vi "Read acquisition start time (0.0 s).vi"(8 "error in (no error)":errorcluster, 11 "Configure Acquisition Record Msg in":refnum<class "Configure Acquisition Record Msg.lvclass">) -> (0 "error out":errorcluster, 2 "acquisition start time (0.0 s)":dbl[unit] format="%.3f", 3 "Configure Acquisition Record Msg out":refnum<class "Configure Acquisition Record Msg.lvclass">)   [LabVIEW 2015, in "CS++Scope.lvlib" / "Configure Acquisition Record Msg.lvclass"]
uses:
  Configure Acquisition Record Msg.lvclass
  Configure Acquisition Record Msg.lvclass/Configure Acquisition Record Msg.ctl
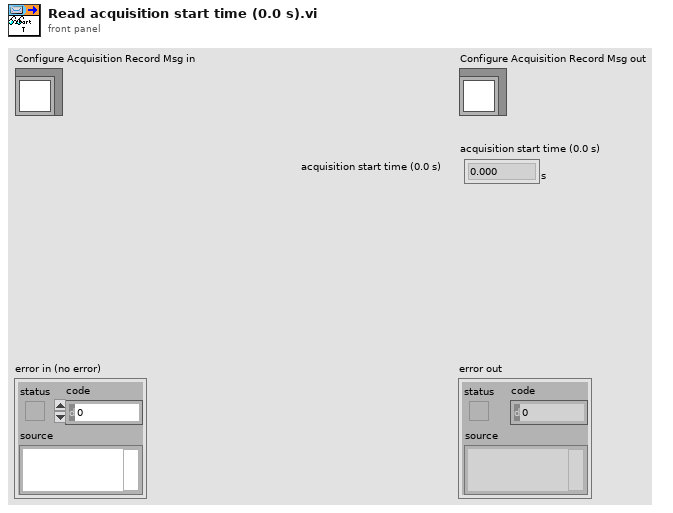
[diagram p1: front panel]
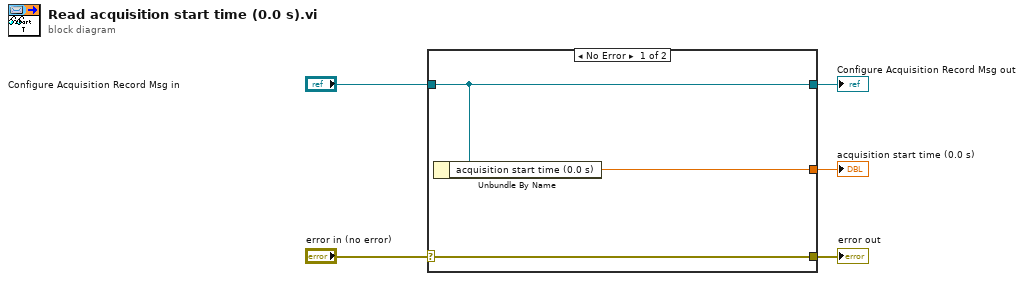
[diagram p0: block diagram]
diagram:
  n1 = case shown="No Error" "error in (no error)" {
    selector: "error in (no error)" -> [w8 w9]
    tunnel: [w8 w9] -> w4
    tunnel: [w7 w10] -> w2
    tunnel: "Configure Acquisition Record Msg in" -> [w7 w10]
    tunnel: [w6 _] -> w1
    frame No Error {
      n2 = Unbundle By Name(w7) -> ("acquisition start time (0.0 s)"=w6:dbl[unit])
    }
    frame Error {
    }
  }
  "error out" <- w4
  "Configure Acquisition Record Msg out" <- w2
  "acquisition start time (0.0 s)" <- w1
